vi "Get Camera Event Status.vi"(11 "camStatus":u32) -> (2 "function return":u32, 3 "camStatus out":u32)   [LabVIEW 2018, in "Copy of Andor SDK.lvlib"]
doc: "EXPNETTYPE unsigned int WINAPI GetCameraEventStatus(DWORD * camStatus);"
uses:
  Copy of Andor SDK.lvlib
  <userlib>/Andor SDK/ATMCD32D.dll
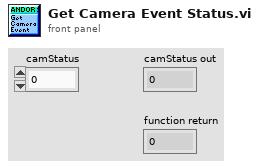
[diagram p1: front panel]
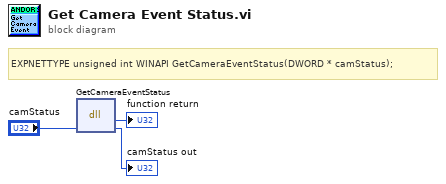
[diagram p0: block diagram]
diagram:
  # "EXPNETTYPE unsigned int WINAPI GetCameraEventStatus(DWORD * camStatus);"
  n1 = dll-call lib="C:/Program Files (x86)/National Instruments/LabVIEW 2018/user.lib/Andor SDK/ATMCD32D.*" fn="GetCameraEventStatus"("camStatus"="camStatus") -> (→"function return":u32, "camStatus"=→"camStatus out":u32)  [unwired: 3 in, 2 out]
